vi "Acquire Host Key Refnum.vi"(8 "error in (no error)":errorcluster, 11 "host key":T1) -> (0 "error out":errorcluster, 2 "libssh2_knownhost*":u64)   [LabVIEW 2013, in "libssh2.lvlib"]
uses:
  libssh2.lvlib
  Host Key Refnum.ctl
  <vilib>/Utility/semaphor.llb/Acquire Semaphore.vi
  Read Host Key Database Refnum.vi
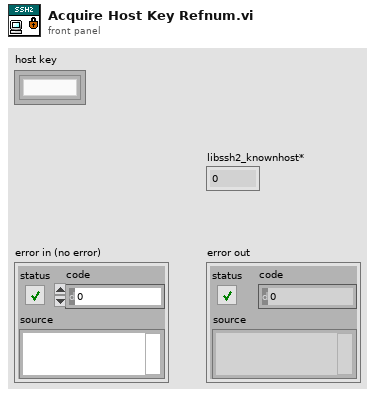
[diagram p1: front panel]
types:
  T1 = typedef "libssh2.lvlib/Host Key Refnum.ctl" = refnum<k1>
  T2 = typedef "libssh2.lvlib/Host Key Database Refnum.ctl" = refnum<k1>
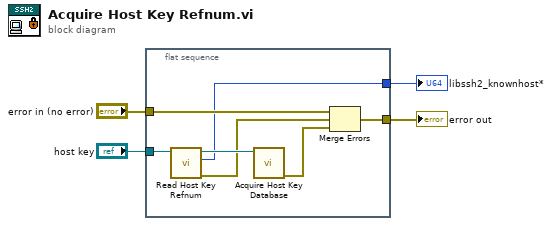
[diagram p0: block diagram]
diagram:
  n1 = flat-sequence {
    tunnel: [w8] -> w4
    tunnel: "error in (no error)" -> [w7]
    tunnel: "host key" -> [w6]
    tunnel: [w5] -> w1
    frame #0 {
      n2 = call "Read Host Key Refnum.vi"("host key"=w6) -> ("error out"=w10:errorcluster, "libssh2_knownhost*"=w5:u64, "host key database"=w11:T2)  [unwired: 8 in]
      n3 = call "Acquire Host Key Database.vi"("host key database"=w11) -> ("error out"=w9:errorcluster)  [unwired: 9 in, 1 out]
      n4 = Merge Errors(w7, w10, w9) -> (w8:errorcluster)
    }
  }
  "error out" <- w4
  "libssh2_knownhost*" <- w1
